vi "1b_Thermometer(170382)(170307).vi"(1 "Temp unit":bool=TRUE) -> (0 "Temperature":sgl(slide)=20.458984 scale=0.0..100.0)   [LabVIEW 2015]
panel:
  out "Temperature Chart":dbl(graph)=20.458984375
  in  "Temperature channel":tag="Dev1/ai0"
  in  "stop":bool
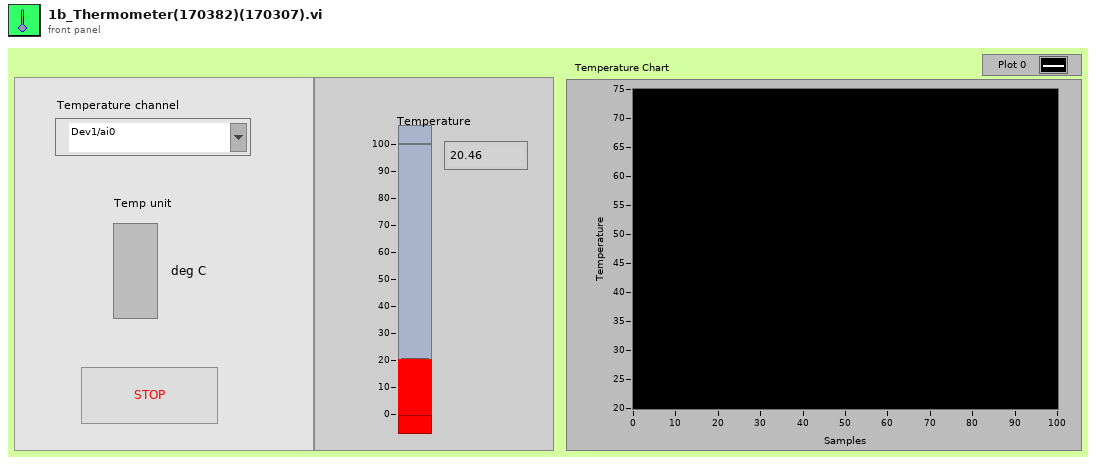
[diagram p1: front panel]
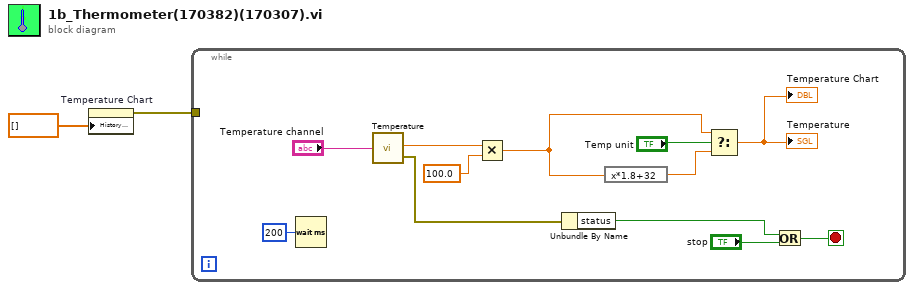
[diagram p0: block diagram]
diagram:
  n1 = property on="Temperature Chart" class="WFChart (strict)"("History Data"=dbl[] []) -> (error out=w1:errorcluster)  [unwired: 2 in, 1 out]
  n2 = while {
    tunnel: w1 -> [_]
    stop <- w11 stop-if-true
    n3 = Wait (ms)(milliseconds to wait=u32 200) -> ()  [unwired: 1 out]
    n4 = call "Temperature.vi"("physical channels"="Temperature channel") -> ("data"=w9:dbl, "error out"=w7:errorcluster)
    n5 = Multiply(x=w9, y=sgl 100.0) -> (x*y=w4:dbl)
    n6 = Unbundle By Name(w7) -> ("status"=w10:bool)
    n7 = expression code="x*1.8+32"(w4) -> (w3:dbl)
    n8 = Select(t=w4, s="Temp unit", f=w3) -> (s? t:f=→"Temperature" →"Temperature Chart":dbl)
    n9 = Or(x=w10, y="stop") -> (x .or. y?=w11:bool)
  }
